vi "TestLocalizeVIs.vi"(8 "error in (no error)":errorcluster) -> (0 "error out":errorcluster)   [LabVIEW 2017]
uses:
  <vilib>/addons/_JKI Toolkits/Caraya/classes/Test/Test.lvclass
  <vilib>/addons/_JKI Toolkits/Caraya/classes/Assert/Assert.lvclass
  src/API/JKI Simple Localization.lvlib
panel:
  # "See block diagram for unit tests of LocalizeVIs.vi"
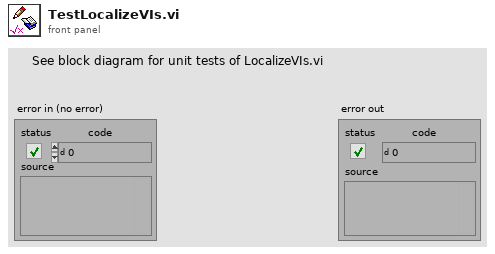
[diagram p1: front panel]
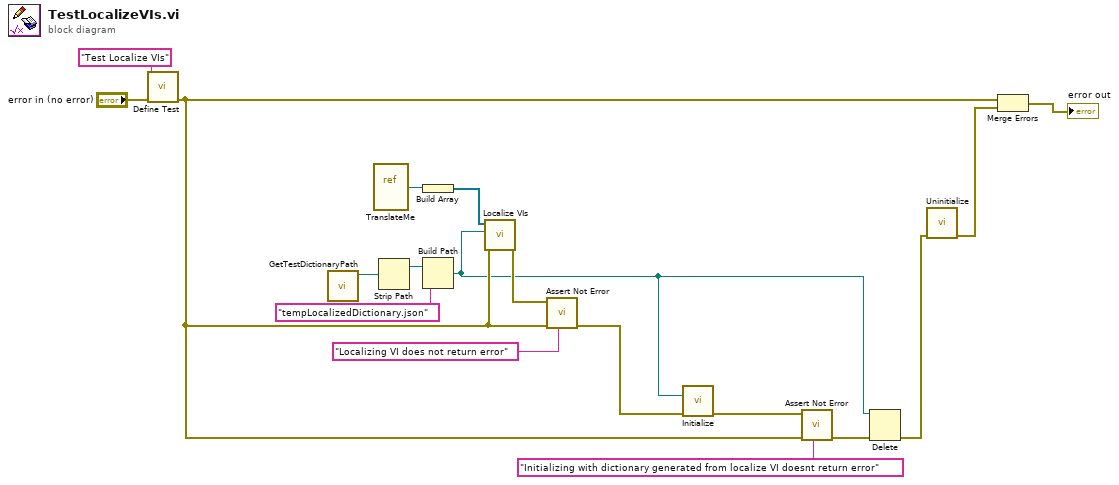
[diagram p0: block diagram]
diagram:
  n1 = call <vilib>:"Define Test.vi"("error in (no error)"="error in (no error)", "Label (VI Title)"="Test Localize VIs") -> ("error out"=w6:errorcluster)  [unwired: 9 in]
  n2 = call "GetTestDictionaryPath.vi"() -> ("Test Dictionary Path"=w13:path)  [unwired: 11 in]
  n3 = vi-ref "TranslateMe.vi"() -> (w10:refnum<vi>)
  n4 = Strip Path(path=w13) -> (stripped path=w12:path)  [unwired: 1 out]
  n5 = Build Array(w10) -> (w9:refnum<vi>[])
  n6 = Build Path(base path=w12, name or relative path="tempLocalizedDictionary.json") -> (appended path=w4:path)
  n7 = call "Localize VIs.vi"("error in (no error)"=w6, "Dictionary Path"=w4, "VIs in"=w9) -> ("error out"=w8:errorcluster)  [unwired: 8 in]
  n8 = call <vilib>:"Assert Not Error.vi"("Label"="Localizing VI does not return error", "error in (no error)"=w6, "Not Error?"=w8) -> ("error out"=w2:errorcluster)  [unwired: 8 in]
  n9 = call "Initialize.vi"("Dictionary File Path"=w4, "error in"=w2) -> ("error out"=w7:errorcluster)  [unwired: 10 in, 3 out]
  n10 = call <vilib>:"Assert Not Error.vi"("Label"="Initializing with dictionary generated from localize VI doesnt return error", "error in (no error)"=w6, "Not Error?"=w7) -> ("error out"=w3:errorcluster)  [unwired: 8 in]
  n11 = Delete(path (use dialog)=w4, error in=w3) -> (error out=w1:errorcluster)  [unwired: 3 in, 2 out]
  n12 = call "Uninitialize.vi"("error in"=w1) -> ("error out"=w14:errorcluster)  [unwired: 10 in]
  n13 = Merge Errors(w6, w14) -> (→"error out":errorcluster)
